vi "Peak Detection and Display.vi"() -> ()   [LabVIEW 2020]
doc: "Demonstrates the use of the Peak Detector VI."
uses:
  <vilib>/Analysis/3filter.llb/Elliptic Filter (DBL).vi
  <vilib>/Analysis/NI_AALBase.lvlib
  <vilib>/Analysis/NI_AAL_SigProc.lvlib
panel:
  in  "signal source":u16(ring) items=["Filtered Noise", "EKG", "Sinc", "Sin + Cos"]
  in  "EKG Mode":i16(ring) items=["static"=0, "scrolling"=-2]
  out "valleys found":i32
  in  "Stop":bool
  in  "filter order":i32=2
  in  "noise seed":i32=1
  in  "peak detector width":i32=3 min=3
  out "Signal Plot":cluster{"Locations":dbl[], "Amplitudes":dbl[]}[](graph)
  out "peaks found":i32
  # "Overview: Demonstrates the use of the Peak Detector VI to find peaks and valleys in a variety of signals.\nRequirements: LabVIEW Full Development System\nInstructions:\n1. Run the VI.\n2. Within the Signal Plot, move the horizontal cursors to adjust the peak detector threshold levels (red for Peaks, blue for Valleys).\n3. Change the signal source along with the noise seed, filter order, and EKG mode to modify the signal shape.\n4. Change the peak detector width to observe how smoothing increases with width.\n5. Click Stop to stop the VI."
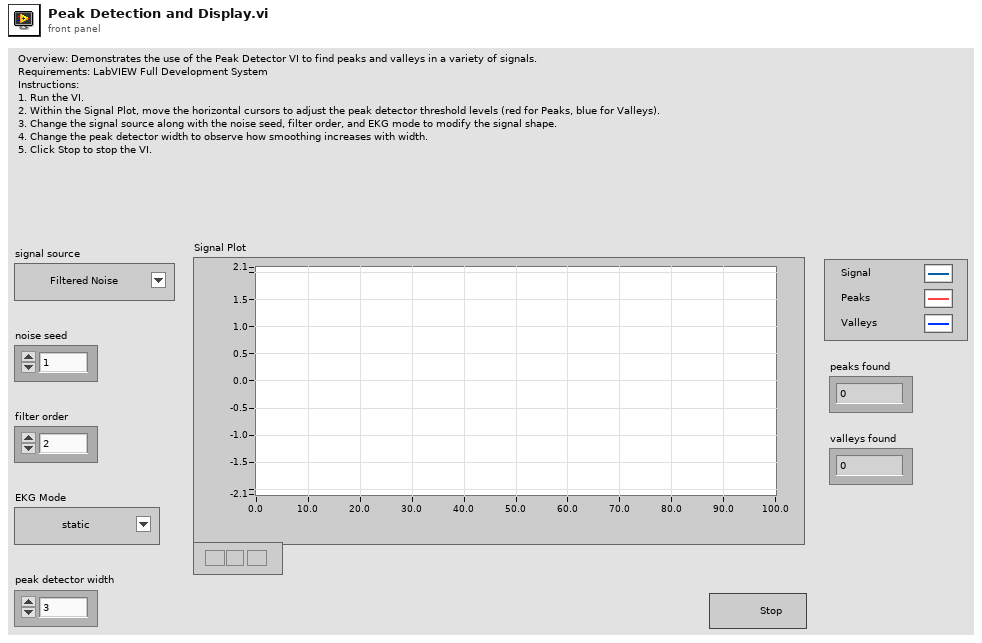
[diagram p1: front panel]
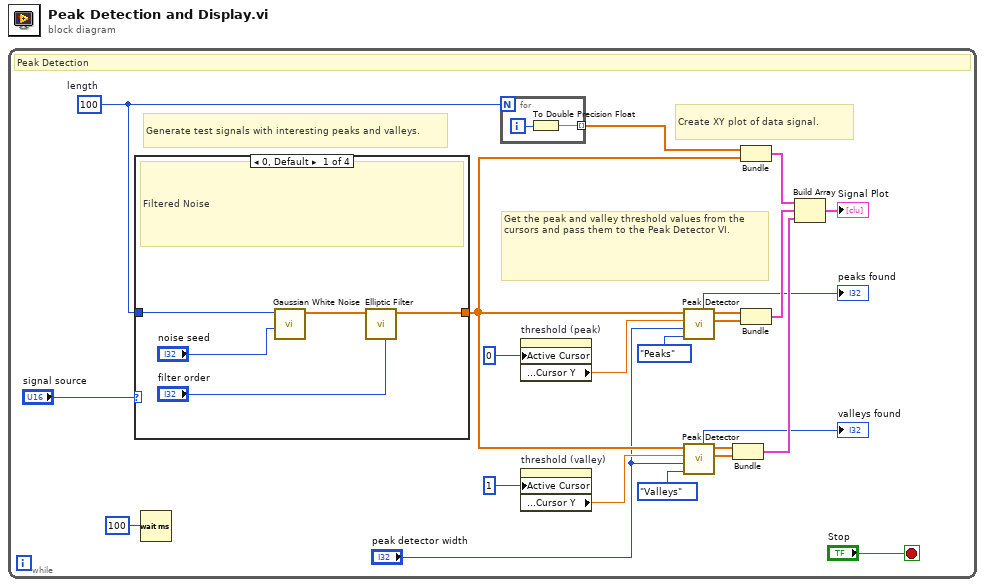
[diagram p0: block diagram]
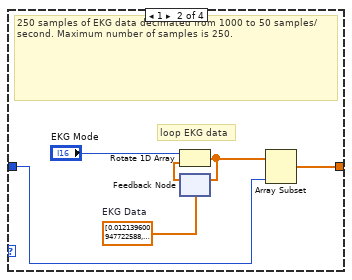
[diagram p2: hidden frame]
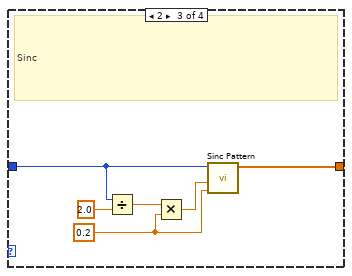
[diagram p3: hidden frame]
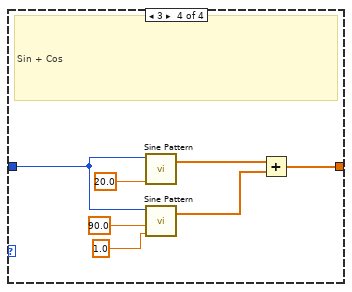
[diagram p4: hidden frame]
diagram:
  n1 = while {
    stop <- "Stop" stop-if-true
    w10 = 100  # length
    # "Get the peak and valley threshold values from the cursors and pass them to the Peak Detector VI."
    # "Create XY plot of data signal."
    # "Generate test signals with interesting peaks and valleys."
    # "Peak Detection"
    n2 = case shown="0, Default" "signal source" {
      tunnel: [w28 w36 w40 w48] -> w9
      tunnel: w10 -> [w30 w32 w39 w46]
      frame 0, Default {
        # "Filtered Noise"
        n3 = call <vilib>:"Gaussian White Noise.vi"("seed"="noise seed", "samples"=w30) -> ("Gaussian noise pattern"=w29:dbl[])  [unwired: 8 in, 1 out]
        n4 = call-poly <vilib>:"Elliptic Filter.vi"("order"="filter order", "X"=w29) -> ("Filtered X"=w28:dbl[])  [unwired: 8 in, 1 out]
      }
      frame 1 {
        w34 = dbl[] [0.012139600947722588, 0.1204944965455566, 0.11889921462709216, 0.0800676634413639, 0.09372867100811462, 0.1215903704395262, 0.10446540283230497, 0.07141030778065277, 0.0843634500592836, 0.10940433857267869, 0.09273506116544213, 0.07435429846089882, 0.17775302501513765, 0.3065686633290967, 0.36418401302282666, 0.27412672045928566, 0.14449726901625132, 0.06402296548891047, 0.055474444161153616, 0.036100325878590446, 0.1186770286983259, 0.3537788154063599, 0.7982020830719359, -1.2269635452787593, -1.5413175167950741, -1.1729876334347535, -0.35411772293599414, -0.07709706053231465, -0.027304988005505383, 0.030060377324908433, 0.07797012817284005, 0.09901072192959604, 0.18523179705138154, 0.35758751077126, 0.5184197582952483, 0.5914729641546187, 0.5881276006820187, 0.5334027735288737, 0.4000013259625401, 0.24498720604258456, 0.1458371502271652, 0.13997617606340304, 0.14767861503410723, 0.12173808129209032, 0.08126736054481143, 0.09932121934746803, 0.11289941003194186, 0.09423081006196077, 0.06765936667047498, 0.08144460506740725, 0.11899963103077821, 0.10867237606099989, 0.08101220897689525, 0.09434750400747845, 0.12229658482075328, 0.16449839075468672, 0.2313259344175102, 0.34852970172486797, 0.37141114350400845, 0.26022986119231767, 0.05719360875627175, 0.03732958784172537, 0.061429953540132795, 0.115384728900427, 0.14666794784015244, 1.0540483974711796, -0.6574183673518581, -1.5474732379921396, -1.3816012201633534, -0.6667176276712435, -0.07235686410159782, -0.00721548416778123, -0.012068120297645932, 0.032007383462091775, 0.11152401638319857, 0.20218059548719458, 0.2855617623145412, 0.4409098532275056, 0.6035721226643459, 0.6498083231847818, 0.5655429141132404, 0.4074244349653328, 0.3074689410313418, 0.2054616609690386, 0.12559533092785613, 0.0880324743499734, 0.11422323625848217, 0.12263782256269917, 0.09136834735481673, 0.05723501679166613, 0.09299409949796553, 0.09084355507250896, 0.07145517675232192, 0.04935876873506096, 0.08438436311447828, 0.0989535482728559, 0.07748106251639456, 0.05177859857719881, 0.10972769160993179, 0.24365500858390168, 0.31430147554801174, 0.3352544281444049, 0.2597936734891093, 0.10654876514286304, 0.04058529973332259, 0.011781491238901445, 0.03817012668473157, 0.13215170347222957, 0.8107840876208048, 0.09723914989779585, -1.489035526096676, -1.4311754367503293, -0.9612908893435409, -0.21818698518563864, -0.049950933650532735, 0.019983913442407034, 0.032152606988631975, 0.046360109431709096, 0.12825344426803828, 0.25758898600174795, 0.417905407292422, 0.5139627867620751, 0.5974008689763063, 0.5951020924923884, 0.4653035110327925, 0.2821972404717557, 0.1633546469126564, 0.1260503434728758, 0.08409405738289659, 0.03720027641482144, 0.020074443785027013, 0.05998916696972105, 0.05972290327720708, 0.028394399802324867, 0.016502538187863725, 0.04068339168224359, 0.041741795070875956, 0.017678106146857425, 0.016553348311421228, 0.04002888294471562, 0.05859619391460098, 0.03933293860667989, 0.13018291946327654, 0.23859231620690902, 0.33386117943181703, 0.21895340269514094, 0.04383697812954624, -0.0019538941761620427, -0.007995740551313767, -0.03628693607678547, 0.035667077113042484, 0.5548085312111103, 0.37696083053978124, -1.4976023978629363, -1.5756884852658988, -1.1259863591370798, -0.30656113137791974, -0.12190409106155943, -0.08058599907930383, -0.017400483123856843, 0.028617965124548755, 0.06566040398981514, 0.15308904252008085, 0.3245829594307986, 0.493594501570732, 0.5501793884505473, 0.5243557994913506, 0.4338191970032014, 0.2679409074135744, 0.1134703921540636, 0.021583960661196583, 0.002969619623208085, 0.010333978368852043, -0.020954446616158223, -0.031574311202989806, -0.010423339355604033, 0.0005819750762649851, -0.013306671911900185, -0.04911904096467989, -0.02355247976487158, -0.0032734061885268863, -0.027881632856645328, -0.041364079223904004, -0.0262107952740536, 0.003597191115312676, 0.059470440649424236, 0.13475605807036575, 0.2327133071812627, 0.20999715366097033, 0.07302369794864476, -0.0756878352464832, -0.06274026045183469, -0.041856972457285674, 0.009173438041878996, 0.26428395677782296, 0.6671163305283284, -1.2806780201956116, -1.6020468559588432, -1.3193715372297998, -0.49274363077386196, -0.13768947466565695, -0.10249186851908754, -0.10244273013629504, -0.060563561959919694, 0.04151234991341134, 0.1243284494208641, 0.23912801221592306, 0.4118750568485528, 0.5521483477976912, 0.5313632070535855, 0.3807827412060248, 0.23835384833413317, 0.13492294965458032, 0.02670344305096497, -0.045512841141119274, -0.0506396372495488, -0.004291991184884786, -0.025208717116017004, -0.06061674115622873, -0.04230259221072288, -0.028099876702536906, -0.041760134434174735, -0.0765383196610732, -0.053595149113861706, -0.02343761827192735, -0.051286651450090856, -0.07758045744889752, -0.07132165108083033, 0.007821664638855164, 0.11363027919848598, 0.17739765826457624, 0.15744478650080235, 0.06121493296301146, -0.09137661413912315, -0.14419901875082705, -0.13048675656883854, -0.03265021203537061, 0.054847703267058186, 0.8534907081956445, -1.026235595903266, -1.6473974782801346, -1.445251070780656, -0.6989098323465748, -0.1996289703384697, -0.11388157997299353, -0.10908018290816052, -0.09649543196259024, -0.012856054404186216, 0.10170783714089084, 0.2323721633256582]  # EKG Data
        # "loop EKG data"
        # "250 samples of EKG data decimated from 1000 to 50 samples/second. Maximum number of samples is 250."
        n5 = feedback #1(w34) -> (w35:dbl[])
        n6 = Rotate 1D Array(1:w35, 2:"EKG Mode") -> (0:w33:dbl[])
        n7 = feedback-in #1(w33) -> ()
        n8 = Array Subset(array=w33, length=w32) -> (w36:dbl[])  [unwired: 1 in]
      }
      frame 2 {
        w37 = 0.2
        # "Sinc"
        n9 = Divide(x=w39, y=2.0) -> (x/y=w42:dbl)
        n10 = Multiply(x=w42, y=w37) -> (x*y=w41:dbl)
        n11 = call <vilib>:"Sinc Pattern.vi"("delta t"=w37, "delay"=w41, "samples"=w39) -> ("Sinc Pattern"=w40:dbl[])  [unwired: 1 in, 1 out]
      }
      frame 3 {
        # "Sin + Cos"
        n12 = call <vilib>:"Sine Pattern.vi"("cycles"=20.0, "samples"=w46) -> ("Sinusoidal Pattern"=w49:dbl[])  [unwired: 2 in, 1 out]
        n13 = call <vilib>:"Sine Pattern.vi"("cycles"=1.0, "phase(degrees)"=90.0, "samples"=w46) -> ("Sinusoidal Pattern"=w47:dbl[])  [unwired: 1 in, 1 out]
        n14 = Add(x=w49, y=w47) -> (x+y=w48:dbl[])
      }
    }
    n15 = Wait (ms)(milliseconds to wait=u32 100) -> ()  [unwired: 1 out]
    n16 = for {
      N: w10 -> [_]
      tunnel: [w24] -> w11 mode=indexing
      i -> [w25]
      n17 = To Double Precision Float(number=w25) -> (double precision float=w24:dbl)
    }
    n18 = property on="threshold (peak)" class="XYGraph (strict)"("Active Cursor"=u32 0) -> ("Cursor.Cursor Position:Cursor Y"=w8:dbl)  [unwired: 2 in, 2 out]
    n19 = property on="threshold (valley)" class="XYGraph (strict)"("Active Cursor"=u32 1) -> ("Cursor.Cursor Position:Cursor Y"=w7:dbl)  [unwired: 2 in, 2 out]
    n20 = call <vilib>:"Peak Detector.vi"("peaks/valleys"=enum32{"Peaks", "Valleys"}."Peaks", "width"="peak detector width", "threshold"=w8, "X"=w9) -> ("Amplitudes"=w21:dbl[], "Locations"=w13:dbl[], "# found"=→"peaks found":i32)  [unwired: 3 in, 2 out]
    n21 = call <vilib>:"Peak Detector.vi"("peaks/valleys"=enum32{"Peaks", "Valleys"}."Valleys", "width"="peak detector width", "threshold"=w7, "X"=w9) -> ("Amplitudes"=w18:dbl[], "Locations"=w19:dbl[], "# found"=→"valleys found":i32)  [unwired: 3 in, 2 out]
    n22 = Bundle("Locations"=w19, "Amplitudes"=w18) -> (w16:cluster{"Locations":dbl[], "Amplitudes":dbl[]})  [unwired: 1 in]
    n23 = Bundle(w11, "Sinc Pattern"=w9) -> (w23:cluster{dbl[], "Sinc Pattern":dbl[]})  [unwired: 1 in]
    n24 = Bundle("Locations"=w13, "Amplitudes"=w21) -> (w20:cluster{"Locations":dbl[], "Amplitudes":dbl[]})  [unwired: 1 in]
    n25 = Build Array(w23, w20, w16) -> (→"Signal Plot":cluster{"Locations":dbl[], "Amplitudes":dbl[]}[])
  }
